vi "MFC WR selective.vi"() -> ()   [LabVIEW 2014]
panel:
  out "Overall Time":u32
  out "Timings":u32[](array[numeric])
  out "MFC PV":u8[](array[numeric])
  out "MFC out":u8[](array[numeric])
  in  "Out Array":u8[](array[numeric])=[65, 48, 48, 48, 48, 48, 13, 65, 48, 48, 48, 48, 48, 13, 67, 48, 48, 48, 48, 48, 13, 68, 48, 48, 48, 48, 48, 13, 69, 48, 48, 48, 48, 48, 13, 70, 48, 48, 48, 48, 48, 13, 71, 48, 48, 48, 48, 48, 13, 72, 48, 48, 48, 48, 48, 13, 73, 48, 48, 48, 48, 48, 13]
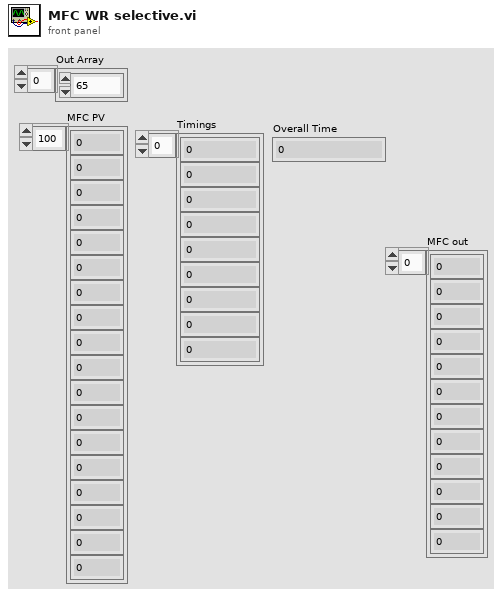
[diagram p1: front panel]
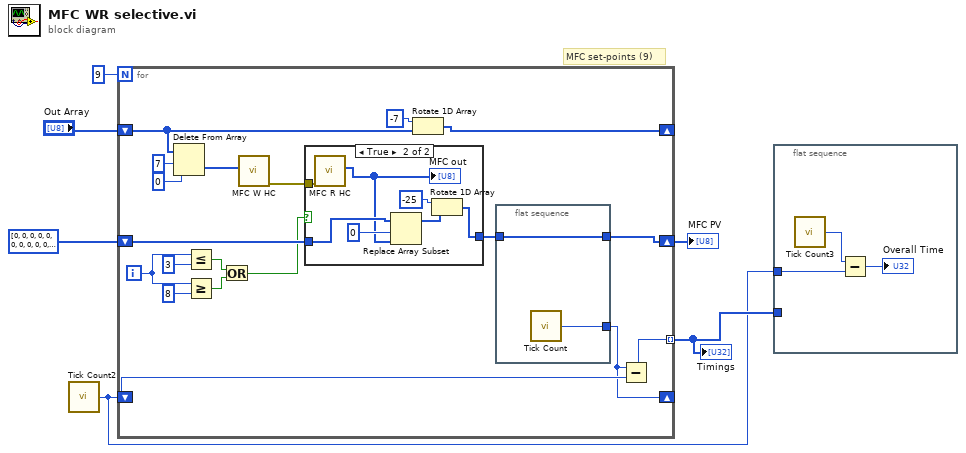
[diagram p0: block diagram]
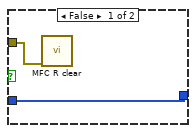
[diagram p2: hidden frame]
diagram:
  # "MFC set-points (9)"
  n1 = call "Tick Count2"() -> ("Tick Count(Ticks)"=w1:u32)
  n2 = for {
    N: 9 -> [_]
    shift-right: [w23] -> _
    shift-left: "Out Array" -> [w24]
    shift-right: [w9] -> w3
    shift-left: u8[] [0, 0, 0, 0, 0, 0, 0, 0, 0, 0, 0, 0, 0, 0, 0, 0, 0, 0, 0, 0, 0, 0, 0, 0, 0, 0, 0, 0, 0, 0, 0, 0, 0, 0, 0, 0, 0, 0, 0, 0, 0, 0, 0, 0, 0, 0, 0, 0, 0, 0, 0, 0, 0, 0, 0, 0, 0, 0, 0, 0, 0, 0, 0, 0, 0, 0, 0, 0, 0, 0, 0, 0, 0, 0, 0, 0, 0, 0, 0, 0, 0, 0, 0, 0, 0, 0, 0, 0, 0, 0, 0, 0, 0, 0, 0, 0, 0, 0, 0, 0, 0, 0, 0, 0, 0, 0, 0, 0, 0, 0, 0, 0, 0, 0, 0, 0, 0, 0, 0, 0, 0, 0, 0, 0, 0] -> [w18]
    tunnel: [w16] -> w2 mode=indexing
    shift-right: [w7] -> _
    shift-left: w1 -> [w17]
    i -> [w10]
    n3 = Delete From Array(array=w24, length=7, index=0) -> (deleted portion=w19:u8[])  [unwired: 1 out]
    n4 = Less Or Equal?(x=w10, y=3) -> (x <= y?=w15:bool)
    n5 = Greater Or Equal?(x=w10, y=8) -> (x >= y?=w14:bool)
    n6 = Or(x=w15, y=w14) -> (x .or. y?=w13:bool)
    n7 = call "MFC W HC.vi"("Byte array"=w19) -> ("error out"=w20:errorcluster)  [unwired: 10 in]
    n8 = case shown="True" w13 {
      tunnel: w20 -> [w28 w36]
      tunnel: w18 -> [w29 w35]
      tunnel: [w29 w32] -> w8
      frame False {
        n9 = call "MFC R clear.vi"("error in"=w28) -> ()  [unwired: 9 in, 1 out]
      }
      frame True {
        n10 = call "MFC R HC.vi"("error in"=w36) -> ("MFC out"=w30:u8[])  [unwired: 8 in, 1 out]
        "MFC out" <- w30
        n11 = Replace Array Subset(array=w35, new element=w30, index=0) -> (w33:u8[])
        n12 = Rotate 1D Array(1:w33, 2:-25 ("n")) -> (0:w32:u8[])
      }
    }
    n13 = Rotate 1D Array(1:w24, 2:-7 ("n")) -> (0:w23:u8[])
    n14 = flat-sequence {
      tunnel: [w27] -> w9
      tunnel: w8 -> [w27]
      tunnel: [w26] -> w7
      frame #0 {
        n15 = call "Tick Count"() -> ("Tick Count(Ticks)"=w26:u32)
      }
    }
    n16 = Subtract(x=w7, y=w17) -> (x-y=w16:u32)
  }
  "MFC PV" <- w3
  "Timings" <- w2
  n17 = flat-sequence {
    tunnel: w2 -> [_]
    tunnel: w1 -> [w37]
    frame #0 {
      n18 = call "Tick Count3"() -> ("Tick Count(Ticks)"=w38:u32)
      n19 = Subtract(x=w38, y=w37) -> (x-y=→"Overall Time":u32)
    }
  }
